vi "Table Configuration Constructor.vi"   [LabVIEW 2020, in "Table.lvlib"]
uses:
  Table.lvlib
  Configuration/Table Configuration Basic DB/Table Configuration Basic DB.lvclass
  Configuration/Table Configuration Adv Schema DB/Table Configuration Adv Schema DB.lvclass
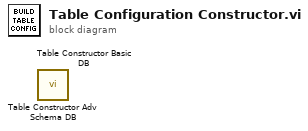
[diagram p0: block diagram]
diagram:
  n1 = call "Table Constructor Adv Schema DB.vi"() -> ()  [unwired: 10 in, 2 out]
  n2 = call "Table Constructor Basic DB.vi"() -> ()  [unwired: 10 in, 2 out]
